vi "Get Nth Serial Port.vi"(0 "N 1..63":i32=1 min=1 max=63 step=1, 7 "error in (no error)":errorcluster) -> (4 "PS Comm Port":refnum<visa-resource-name>, 15 "error out":errorcluster)   [LabVIEW 2025]
doc: "Author: Scott Hannahs <sth@magnet.fsu.edu>\n\nThis software is licensed for use under the “MIT License\"\nCopyright (c) 2025 Scott Hannahs, sth@sth@magnet.sthnet.net\n\nPermission is hereby granted, free of charge, to any person obtaining a copy of this software and associated documentation files (the \"Software\"), to deal in the Software without restriction, including without limitation the rights to use, copy, modify, merge, publish, distribute, sublicense, and/or sell copies of the Software, and to permit persons to whom the Software is furnished to do so, subject to the following conditions: The above copyright notice and this permission notice shall be included in all copies or substantial portions of the Software.\n\nTHE SOFTWARE IS PROVIDED \"AS IS\", WITHOUT WARRANTY OF ANY KIND, EXPRESS OR IMPLIED, INCLUDING BUT NOT LIMITED TO THE WARRANTIES OF MERCHANTABILITY, FITNESS FOR A PARTICULAR PURPOSE AND NONINFRINGEMENT. IN NO EVENT SHALL THE AUTHORS OR COPYRIGHT HOLDERS BE LIABLE FOR ANY CLAIM, DAMAGES OR OTHER LIABILITY, WHETHER IN AN ACTION OF CONTRACT, TORT OR OTHERWISE, ARISING FROM, OUT OF OR IN CONNECTION WITH THE SOFTWARE OR THE USE OR OTHER DEALINGS IN THE SOFTWARE."
panel:
  out "Found":bool
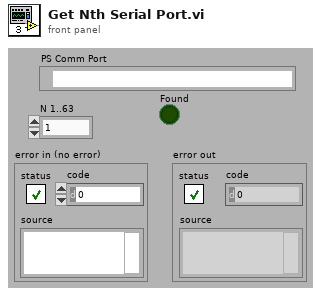
[diagram p1: front panel]
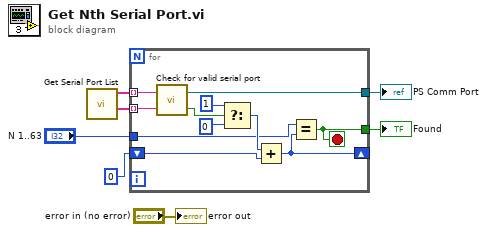
[diagram p0: block diagram]
diagram:
  n1 = call "Get Serial Port List.vi"() -> ("Port Names"=w4:string[], "VISA Name"=w3:string[])  [unwired: 7 in, 3 out]
  n2 = for {
    tunnel: [w17] -> w7
    tunnel: w3 -> [w18] mode=indexing
    tunnel: w4 -> [w16] mode=indexing
    shift-right: [w11] -> _
    shift-left: 0 ("N") -> [w13]
    tunnel: "N 1..63" -> [w10]
    tunnel: [w9] -> w5
    stop <- w9 stop-if-true
    n3 = call "Check for valid serial port.vi"("Serial Port Name"=w16, "PS Communication Port In"=w18) -> ("Valid Serial Port"=w15:bool, "PS Communication Port out"=w17:refnum<visa-resource-name>)
    n4 = Select(t=1 ("N"), s=w15, f=0 ("N")) -> (s? t:f=w14:i32)
    n5 = Add(x=w14, y=w13) -> (x+y=w11:i32)
    n6 = Equal?(x=w10, y=w11) -> (x = y?=w9:bool)
  }
  "PS Comm Port" <- w7
  "Found" <- w5
  "error out" <- "error in (no error)"
